vi "Voltage Measurement.vi"() -> ()   [LabVIEW 2021, in "Main.lvlib"]
uses:
  Main.lvlib
  SMU/SMU.lvlib
  DMM/DMM.lvlib
  Power Measurement/Power Measurement.lvlib
  <instrlib>/niDMM/nidmm.llb/niDMM Resolution in Digits.ctl
panel:
  out "Current Meas":dbl[](array[numeric])
  out "Voltage Meas":dbl[](array[numeric])
  in  "Physical Channel":tag="PowerModule/power"
  in  "Voltage Setpoint":dbl=6.0
  in  "Current Setpoint":dbl=3.0
  in  "Calculate Analysis?":bool
  out "Signal Out of Range":bool
  out "Measurement":dbl format="%.6p"
  in  "Resolution in Digits":T1=5.5 items=["3 1/2"=3.5, "4 1/2"=4.5, "5 1/2"=5.5, "6 1/2"=6.5, "7 1/2"=7.5]
  in  "Range":dbl=10.0 format="%.2f"
  in  "Device Name":refnum<k15>="Dev1"
  out "error out":errorcluster
  out "Current Measurement":dbl
  out "Voltage Measurement":dbl
  in  "error in":errorcluster
  in  "Voltage Level Range":dbl=6.0 format="%.5p"
  in  "Voltage Level":dbl=2.0 format="%.5p"
  in  "Vin SMU Channel":string="0"
  in  "Current Limit Range":dbl=0.01 format="%.3p"
  in  "Current Limit":dbl=0.01 format="%.3p"
  in  "Vin SMU":refnum<k15>="Dev1"
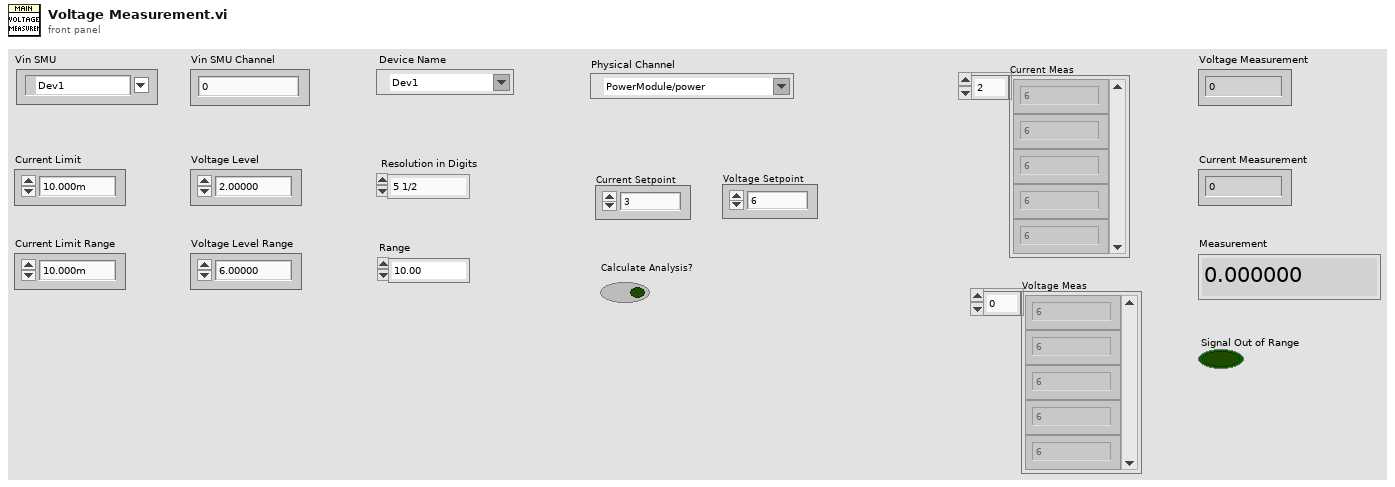
[diagram p1: front panel]
types:
  T1 = typedef "niDMM Resolution in Digits.ctl" = dbl
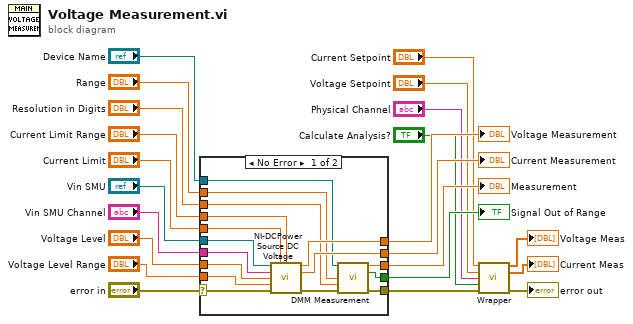
[diagram p0: block diagram]
diagram:
  n1 = case shown="No Error" "error in" {
    selector: "error in" -> [w32 w39]
    tunnel: "Vin SMU" -> [w38 _]
    tunnel: "Current Limit" -> [w37 _]
    tunnel: "Current Limit Range" -> [w36 _]
    tunnel: "Vin SMU Channel" -> [w35 _]
    tunnel: "Voltage Level" -> [w34 _]
    tunnel: "Voltage Level Range" -> [w33 _]
    tunnel: [w31 _] -> w15
    tunnel: [w30 _] -> w14
    tunnel: [w29 w39] -> w2
    tunnel: "Device Name" -> [w27 _]
    tunnel: "Range" -> [w26 _]
    tunnel: "Resolution in Digits" -> [w25 _]
    tunnel: [w24 _] -> w10
    tunnel: [w23 _] -> w9
    frame No Error {
      n2 = call "NI-DCPower Source DC Voltage.vi"("Vin SMU"=w38, "Current Limit"=w37, "Current Limit Range"=w36, "Vin SMU Channel"=w35, "Voltage Level"=w34, "Voltage Level Range"=w33, "error in"=w32) -> ("Voltage Measurement"=w31:dbl, "Current Measurement"=w30:dbl, "error out"=w28:errorcluster)  [unwired: 6 in]
      n3 = call "DMM Measurement.vi"("Device Name"=w27, "Range"=w26, "Resolution in Digits"=w25, "error in"=w28) -> ("Measurement"=w24:dbl, "Signal Out of Range"=w23:bool, "error out"=w29:errorcluster)  [unwired: 9 in]
    }
    frame Error {
    }
  }
  "Voltage Measurement" <- w15
  "Current Measurement" <- w14
  "Measurement" <- w10
  "Signal Out of Range" <- w9
  n4 = call "Wrapper.vi"("Current Setpoint"="Current Setpoint", "Voltage Setpoint"="Voltage Setpoint", "Physical Channel"="Physical Channel", "Calculate Analysis?"="Calculate Analysis?", "error in (no error)"=w2) -> ("voltage"=→"Voltage Meas":dbl[], "Current"=→"Current Meas":dbl[], "error out"=→"error out":errorcluster)  [unwired: 8 in]
